vi "Pairwise_distances.vi"(8 "error in":errorcluster caption="entrée d'erreur", 9 "Y":string[][](array[string]), 10 "X":string[][](array[string]), 11 "pairwise_distances":T2={"metric "="euclidean", "n_jobs"="None", "force_all_finite "="True"}) -> (0 "error out":errorcluster caption="sortie d'erreur", 3 "Data":T1)   [LabVIEW 2020]
doc: "Compute the distance matrix from a vector array X and optional Y.\n\nThis method takes either a vector array or a distance matrix, and returns a distance matrix. If the input is a vector array, the distances are computed. If the input is a distances matrix, it is returned instead.\n\nThis method provides a safe way to take a distance matrix as input, while preserving compatibility with many other algorithms that take a vector array.\n\nIf Y is given (default is None), then the returned matrix is the pairwise distance between the arrays from both X and Y.\n\nValid values for metric are:\n\nFrom scikit-learn: [‘cityblock’, ‘cosine’, ‘euclidean’, ‘l1’, ‘l2’, ‘manhattan’]. These metrics support sparse matrix inputs. [‘nan_euclidean’] but it does not yet support sparse matrices.\n\nFrom scipy.spatial.distance: [‘braycurtis’, ‘canberra’, ‘chebyshev’, ‘correlation’, ‘dice’, ‘hamming’, ‘jaccard’, ‘kulsinski’, ‘mahalanobis’, ‘minkowski’, ‘rogerstanimoto’, ‘russellrao’, ‘seuclidean’, ‘sokalmichener’, ‘sokalsneath’, ‘sqeuclidean’, ‘yule’] See the documentation for scipy.spatial.distance for details on these metrics. These metrics do not support sparse matrix inputs.\n\nNote that in the case of ‘cityblock’, ‘cosine’ and ‘euclidean’ (which are valid scipy.spatial.distance metrics), the scikit-learn implementation will be used, which is faster and has support for sparse matrices (except for ‘cityblock’). For a verbose description of the metrics from scikit-learn, see the __doc__ of the sklearn.pairwise.distance_metrics function.\n\n\n\nParameters : \n\n- X : array [n_samples_a, n_samples_a] if metric == “precomputed”, or, [n_samples_a, n_features] otherwise\nArray of pairwise distances between samples, or a feature array.\n\n- Y : array [n_samples_b, n_features], optional\nAn optional second feature array. Only allowed if metric != “precomputed”.\n\n- metric : string, or callable\nThe metric to use when calculating distance between instances in a feature array. If metric is a string, it must be one of the options allowed by scipy.spatial.distance.pdist for its metric parameter, or a metric listed in pairwise.PAIRWISE_DISTANCE_FUNCTIONS. If metric is “precomputed”, X is assumed to be a distance matrix. Alternatively, if metric is a callable function, it is called on each pair of instances (rows) and the resulting value recorded. The callable should take two arrays from X as input and return a value indicating the distance between them.\n\n- n_jobs : int or None, optional (default=None)\nThe number of jobs to use for the computation. This works by breaking down the pairwise matrix into n_jobs even slices and computing them in parallel.\n\nNone means 1 unless in a joblib.parallel_backend context. -1 means using all processors. See Glossary for more details.\n\n- force_all_finite : boolean or ‘allow-nan’, (default=True)\nWhether to raise an error on np.inf, np.nan, pd.NA in array. The possibilities are:\n\nTrue : Force all values of array to be finite.\n\nFalse : accepts np.inf, np.nan, pd.NA in array.\n\n‘allow-nan’ : accepts only np.nan and pd.NA values in array. Values cannot be infinite.\n\n\nReturns : \n\n- D : array [n_samples_a, n_samples_a] or [n_samples_a, n_samples_b]\nA distance matrix D such that D_{i, j} is the distance between the ith and jth vectors of the given matrix X, if Y is None. If Y is not None, then D_{i, j} is the distance between the ith array from X and the jth array from Y."
uses:
  Pairwise_distances.lvclass
panel:
  out "Pairwise_distances.lvclass":refnum<class "Pairwise_distances.lvclass">
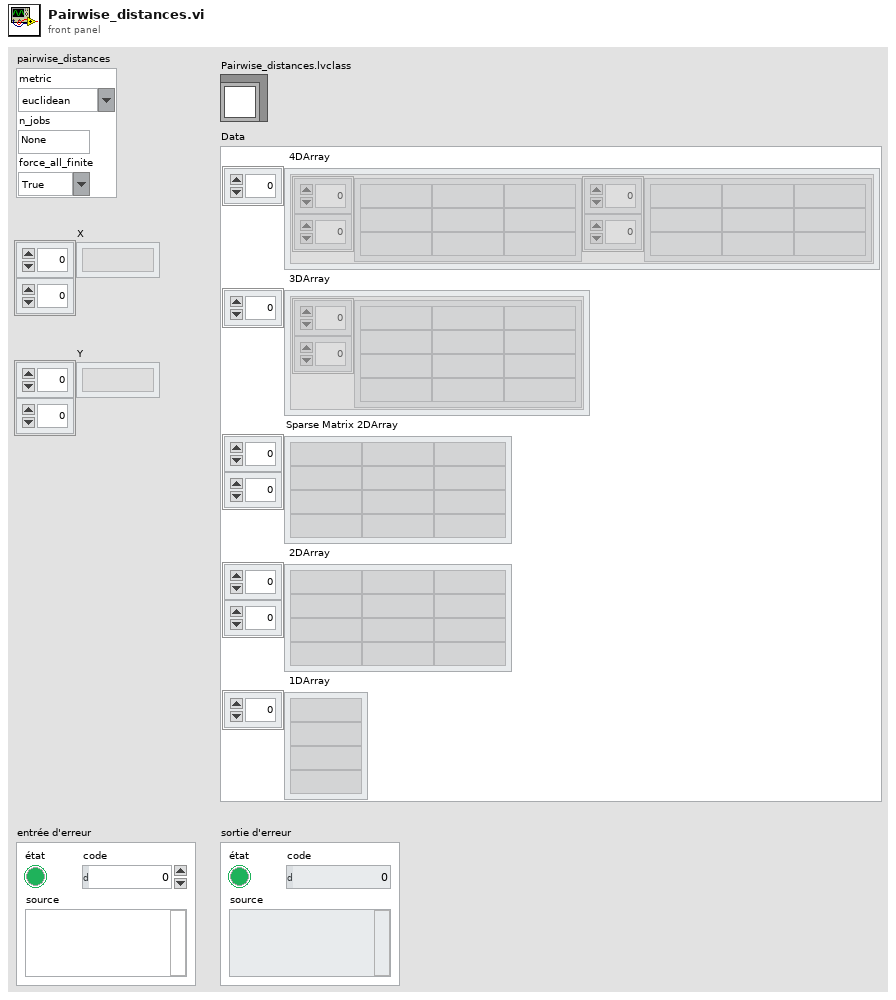
[diagram p1: front panel]
types:
  T1 = cluster{" 4DArray":cluster{"1":string[][], "2":string[][]}[], " 3DArray":cluster{"Tableau":string[][]}[], "Sparse Matrix 2DArray":string[][], " 2DArray":string[][], " 1DArray":string[]}
  T2 = cluster{"metric ":string, "n_jobs":string, "force_all_finite ":string}
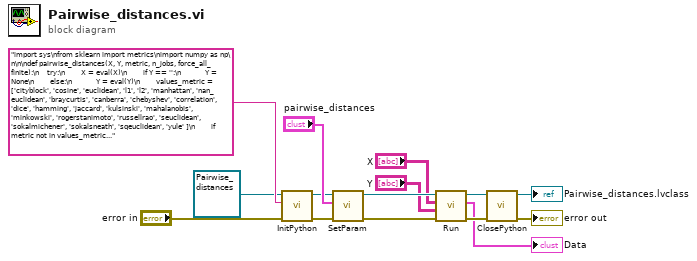
[diagram p0: block diagram]
diagram:
  n1 = call-dynamic "InitPython.vi"("error in (no error)"="error in", "Python Instruction"="import sys\nfrom sklearn import metrics\nimport numpy as np\n\n\ndef pairwise_distances(X, Y, metric, n_jobs, force_all_finite):\n    try:\n        X = eval(X)\n        if Y == '':\n            Y = None\n        else:\n            Y = eval(Y)\n        values_metric = ['cityblock', 'cosine', 'euclidean', 'l1', 'l2', 'manhattan', 'nan_euclidean', 'braycurtis', 'canberra', 'chebyshev', 'correlation', 'dice', 'hamming', 'jaccard', 'kulsinski', 'mahalanobis', 'minkowski', 'rogerstanimoto', 'russellrao', 'seuclidean', 'sokalmichener', 'sokalsneath', 'sqeuclidean', 'yule' ]\n        if metric not in values_metric:\n            metric = eval(metric)\n        if n_jobs == 'None' or n_jobs == '':\n            n_jobs = None\n        else:\n            n_jobs = eval(n_jobs)\n        if force_all_finite == 'True':\n            force_all_finite = True\n        elif force_all_finite == 'False':\n            force_all_finite = False\n        else:\n            pass\n        pairwise_distances = metrics.pairwise.pairwise_distances(X, Y, metric, n_jobs, force_all_finite)\n        pairwise_distances = pairwise_distances.tolist()\n        return str(pairwise_distances)\n    except:\n        erreur = sys.exc_info()\n        typerr = u\"%s\" % (erreur[0])\n        typerr = typerr[typerr.find(\"'\")+1:typerr.rfind(\"'\")]\n        msgerr = u\"%s\" % (erreur[1])\n        message = str('/!\\\\ {0} : {1}'. format(typerr,msgerr))\n        return message", "Scikit-learn en entrée"=refnum<class "Pairwise_distances.lvclass"> refnum ("Pairwise_distances.lvclass")) -> ("error out"=w8:errorcluster, "Scikit-learn en sortie"=w9:refnum<class "Pairwise_distances.lvclass">)  [unwired: 7 in]
  n2 = call-dynamic "SetParam.vi"("error in (no error)"=w8, "pairwise_distances"="pairwise_distances", "Pairwise_distances.lvclass"=w9) -> ()  [unwired: 7 in, 2 out]
  n3 = call-dynamic "Run.vi"("error in (no error)"=w8, "Y"="Y", "X"="X", "Pairwise_distances.lvclass"=w9) -> ("error out"=w6:errorcluster, "Data"=→"Data":T1, "Pairwise_distances.lvclass"=w7:refnum<class "Pairwise_distances.lvclass">)  [unwired: 5 in]
  n4 = call-dynamic "ClosePython.vi"("error in (no error)"=w6, "Scikit-learn en entrée"=w7) -> ("error out"=→"error out":errorcluster, "Scikit-learn en sortie"=→"Pairwise_distances.lvclass":refnum<class "Pairwise_distances.lvclass">)  [unwired: 8 in]
